vi "Create Unit Test.vi"(5 "Unit Test Destination Dir":path=path "C:/Program Files (x86)/National Instruments/LabVIEW 2013/vi.lib/LabVIEW Hacker/VIChallenge/Challenges/Core/Math/Add/Custom Unit Test.lvtest", 7 "User VI":path=path "C:/Program Files (x86)/National Instruments/LabVIEW 2013/vi.lib/LabVIEW Hacker/VIChallenge/Challenges/Core/Math/Add/Add Example.vi", 8 "Error In":errorcluster, 10 "Unit Test Template":path=path "C:/Program Files (x86)/National Instruments/LabVIEW 2013/vi.lib/LabVIEW Hacker/VIChallenge/Challenges/Core/Math/Add/Add Template.lvtest", 11 "Template VI Name":string) -> (0 "Error Out":errorcluster, 2 "Unit Test Template":path=path "C:/Program Files (x86)/National Instruments/LabVIEW 2013/vi.lib/LabVIEW Hacker/VIChallenge/Challenges/Core/Math/Add/Add Template.lvtest")   [LabVIEW 2013, in "VIChallenge.lvlib"]
uses:
  VIChallenge.lvlib
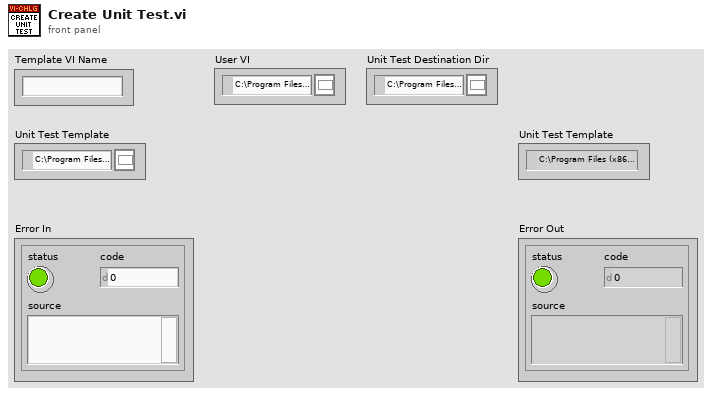
[diagram p1: front panel]
types:
  T1 = enum16{"big-endian, network order", "native, host order", "little-endian"}
  T2 = enum16{"open", "replace", "create", "open or create", "replace or create", "replace or create with confirmation"}
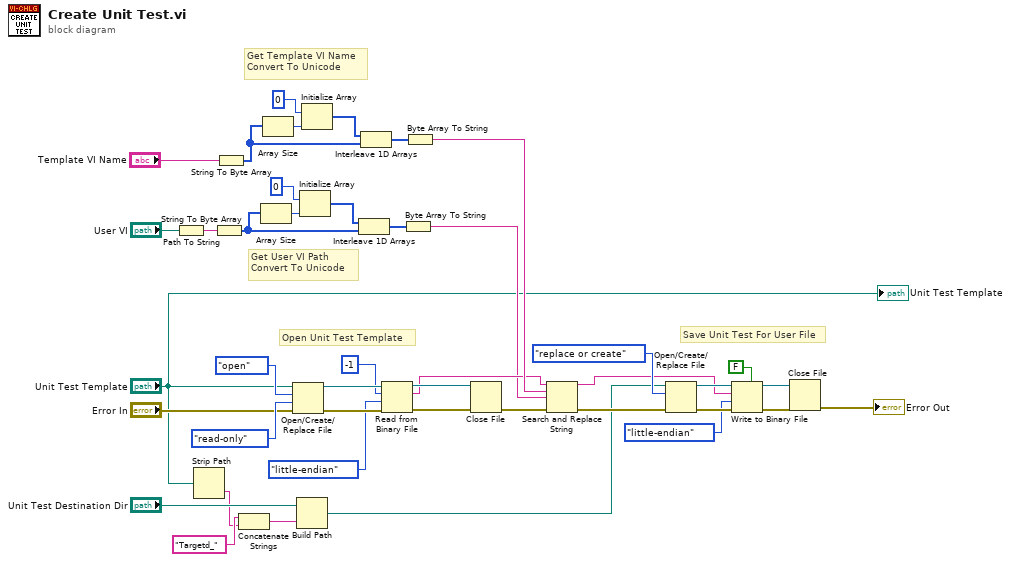
[diagram p0: block diagram]
diagram:
  # "Save Unit Test For User File"
  # "Open Unit Test Template"
  # "Get User VI Path\nConvert To Unicode"
  # "Get Template VI Name\nConvert To Unicode"
  n1 = Path To String(path="User VI") -> (string=w14:string)
  n2 = Strip Path(path="Unit Test Template") -> (name=w2:string)  [unwired: 1 out]
  n3 = String To Byte Array(string=w14) -> (unsigned byte array=w15:u8[])
  n4 = String To Byte Array(string="Template VI Name") -> (unsigned byte array=w41:u8[])
  n5 = Concatenate Strings("Targetd_" ("string"), w2) -> (w1:string)
  n6 = Array Size(array=w15) -> (size(s)=w16:i32)
  n7 = Array Size(array=w41) -> (size(s)=w40:i32)
  n8 = Open/Create/Replace File(file path (use dialog)="Unit Test Template", error in="Error In", operation (0:open)=T2."open", access (0:read/write)=enum16{"read/write", "read-only", "write-only"}."read-only") -> (refnum out=w26:refnum<file>, error out=w27:errorcluster)  [unwired: 2 in, 1 out]
  n9 = Build Path(base path="Unit Test Destination Dir", name or relative path=w1) -> (appended path=w4:path)
  n10 = Initialize Array(u8 0, w16) -> (w18:u8[])
  n11 = Initialize Array(u8 0, w40) -> (w38:u8[])
  n12 = Interleave 1D Arrays(w18, w15) -> (w19:u8[])
  n13 = Interleave 1D Arrays(w38, w41) -> (w37:u8[])
  n14 = Read from Binary File(8:w27, 9:T1."little-endian" ("byte order (0:big-endian, network order)"), 10:-1 ("count (1)"), 11:w26) -> (0:w10:errorcluster, 2:w24:string, 3:w25:refnum<file>)  [unwired: 2 in, 1 out]
  n15 = Byte Array To String(unsigned byte array=w19) -> (string=w13:string)
  n16 = Byte Array To String(unsigned byte array=w37) -> (string=w36:string)
  n17 = Close File(refnum=w25, error in=w10) -> (error out=w9:errorcluster)  [unwired: 1 out]
  n18 = Search and Replace String(input string=w24, search string=w36, replace string=w13, error in=w9) -> (result string=w28:string, error out=w8:errorcluster)  [unwired: 4 in, 2 out]
  n19 = Open/Create/Replace File(file path (use dialog)=w4, error in=w8, operation (0:open)=T2."replace or create") -> (refnum out=w30:refnum<file>, error out=w33:errorcluster)  [unwired: 3 in, 1 out]
  n20 = Write to Binary File(file (use dialog)=w30, data=w28, error in=w33, 5:FALSE ("prepend array or string size? (T)"), 9:T1."little-endian" ("byte order (0:big-endian, network order)")) -> (refnum out=w31:refnum<file>, error out=w32:errorcluster)  [unwired: 1 in, 1 out]
  n21 = Close File(refnum=w31, error in=w32) -> (error out=→"Error Out":errorcluster)  [unwired: 1 out]
  "Unit Test Template" <- "Unit Test Template"
